vi "Process.vi"(8 "error in":errorcluster, 11 "Oxford1820 UI in":refnum<class "Instrument.Oxford1820 UI.lvclass">) -> (0 "error out":errorcluster, 3 "Oxford1820 UI out":refnum<class "Instrument.Oxford1820 UI.lvclass">)   [LabVIEW 2016, in "Instrument.Oxford1820 UI.lvclass"]
doc: "---------------------------------------------------------------\nJKI State Machine Objects™\nhttp://jki.net/state-machine-objects/\nCopyright (C) 2005-2015, JKI <info@jki.net>\nALL RIGHTS RESERVEDJKI State Machine Objects (SMO) 1.0.0.5\nJKI - JKI\nCopyright (c) 2016, JKI"
uses:
  Instrument.Oxford1820 UI.lvclass
  C:/Program Files (x86)/National Instruments/LabVIEW 2016/vi.lib/JKI/JKI SMO/SMO/SMO.lvclass
  C:/Program Files (x86)/National Instruments/LabVIEW 2016/user.lib/LevyLab/Levylab Instruments/SMOs/Instrument UI/Instrument UI.lvclass
  C:/Program Files (x86)/National Instruments/LabVIEW 2016/vi.lib/JKI/JKI SMO/SMO.UI/SMO.UI.lvclass
  <vilib>/JKI/JKI SMO/SMO/Typedefs/Parent Call--Enum.ctl
  Instrument.Oxford1820/Instrument.Oxford1820.lvclass
  C:/Program Files (x86)/National Instruments/LabVIEW 2016/user.lib/LevyLab/Levylab Instruments/SMOs/Instrument/Instrument.lvclass
  <userlib>/LevyLab/Levylab Instruments/SMOs/Instrument UI/Instrument UI.lvclass/Instrument UI.ctl
  Instrument.Oxford1820/Typedefs/getAll.ctl
  Instrument.Oxford1820/Typedefs/Fill Mode-Combo.ctl
  <instrlib>/Mercury iXX/Public/Libraries/Magnet/Controls/Switch Heater.ctl
  <userlib>/LevyLab/Levylab Instruments/SMOs/Instrument/Instrument.lvclass
  <userlib>/LevyLab/Levylab Instruments/SMOs/Instrument UI/Instrument UI.lvclass
  <vilib>/JKI/JKI SMO/SMO/SMO.lvclass
  <vilib>/JKI/JKI SMO/SMO.UI/SMO.UI.lvclass
  <instrlib>/Mercury iXX/Public/Libraries/Magnet.lvlib
panel:
  in  "Open Target":dbl=100.0 format="%.1f (%%)"
  out "System Time (HH:MM:SS)":dbl=165.3592643737793 format="%<%I:%M:%S %p>T"
  out "LPF on":dbl format="%<%H:%M:%S>t"
  out "PS Heat on (HH:MM:SS)":dbl format="%<%H:%M:%S>t"
  out "ETA":dbl=3660699600.0 format="%<%I:%M:%S %p %m/%d/%Y>T"
  out "version":string="v20/10/28"
  out "Waveform Chart 2":T1(graph)
  out "N2 LEVEL":dbl format="%.0f %"
  in  "Window Maximize":bool
  in  "Window Minimize":bool
  out "Magnet Status 3":string="Status: Clamped"
  in  "Remote Mode":bool
  out "Sentinel":bool=TRUE
  out "Voltage Meter":dbl(knob) caption="Voltage (V)" scale=-10.0..10.0
  out "Current Meter":dbl(knob) caption="Voltage (V)" scale=-180.0..180.0
  out "Magnet Field Meter":dbl(knob) caption="Voltage (V)" scale=-20.0..20.0
  in  "Hold":bool
  in  "To Set":bool
  in  "Export":bool
  out "PSU Field":dbl format="%#.5f T"
  in  "Target Field (T)":dbl caption="Field" format="%.2f"
  out "Target Field (T)":dbl caption="Field" format="%.2f T"
  in  "Target Rate (T/min)":dbl=0.1 caption="Rate" min=0.0 max=1.0 format="%.2f"
  out "Target Rate (T/min)":dbl caption="Rate" format="%.2f T/min"
  out "Field":dbl format="%.5f T"
  out "He LEVEL":dbl format="%.0f %"
  in  "PS Heat":bool
  in  "To Zero":bool
  in  "Clamp":bool
  out "N2 LVL":dbl format="%.1f (%%)"
  out "He LVL Chart":dbl(slide)=52.0833 scale=0.0..100.0
  out "N2 LVL Chart":dbl(slide)=61.3025 scale=0.0..100.0
  out "He LVL":dbl format="%.1f (%%)"
  in  "Fast/Slow Fill":bool
  in  "Open Needle Valve":bool
  in  "Close Needle Valve":bool
  in  "LPF Power":bool
  out "Needle Valve":dbl format="%.1f (%%)"
  out "Pressure":dbl format="%_5f mB"
  out "Magnet T":dbl format="%_2f K"
  out "Magnet R":dbl format="%_3f ohms"
  out "Voltage":dbl format="%.5f V"
  out "Current":dbl format="%.5f A"
  out "Magnet Status 2":string="Status: Clamped"
  in  "Power":bool
  # "Obsolete controls?"
  # "Actions"
  # "Targets"
  # "Status"
  # "Slow Rates\nCurrent Range (A)     Field Range (T)  Rate (T/min)\n0       -- 100        0    -- 11.5     0.91\n100     -- 150        11.5 -- 17.2     0.23\n150     -- 155.467    17.2 -- 18       0.11\n155.567 -- 172.471    18   -- 20       0.11\n\nFast Rates\nCurrent Range (A)     Field Range (T)  Rate (T/min)\n0       -- 155.467    0    -- 18       1.0\n155.567 -- 172.471    18   -- 20       0.25"
  # "IPS"
  # "PS Switch"
  # "Level"
  # "Level Graph"
  # "LPF"
  # "Helium"
  # "Nitrogen"
  # "^^^^"
  # "Needle Valve"
  # "Slow Rates\nCurrent Range (A)     Field Range (T)   Rate (T/min)\n0       -- 100        0    -- 11.5      0.91\n100     -- 150        11.5 -- 17.2      0.23\n150     -- 155.467    17.2 -- 18        0.11\n155.567 -- 172.471    18   -- 20        0.11\n\nFast Rates\nCurrent Range (A)     Field Range (T)   Rate (T/min)\n0       -- 155.467    0    -- 18        1.0\n155.567 -- 172.471    18   -- 20        0.25"
  # "SMO UI Template"
  # "For instructions on how to use the JKI State Machine Objects, examples and video tutorials, visit:\nhttp://jki.net/state-machine-objects/\n\nJKI State Machine Objects™\nhttp://jki.net/state-machine-objects/\nCopyright (C) 2005-2015, JKI <info@jki.net>\nALL RIGHTS RESERVED"
  # "Voltage (V)"
  # "Current (A)"
  # "Magnet (T)"
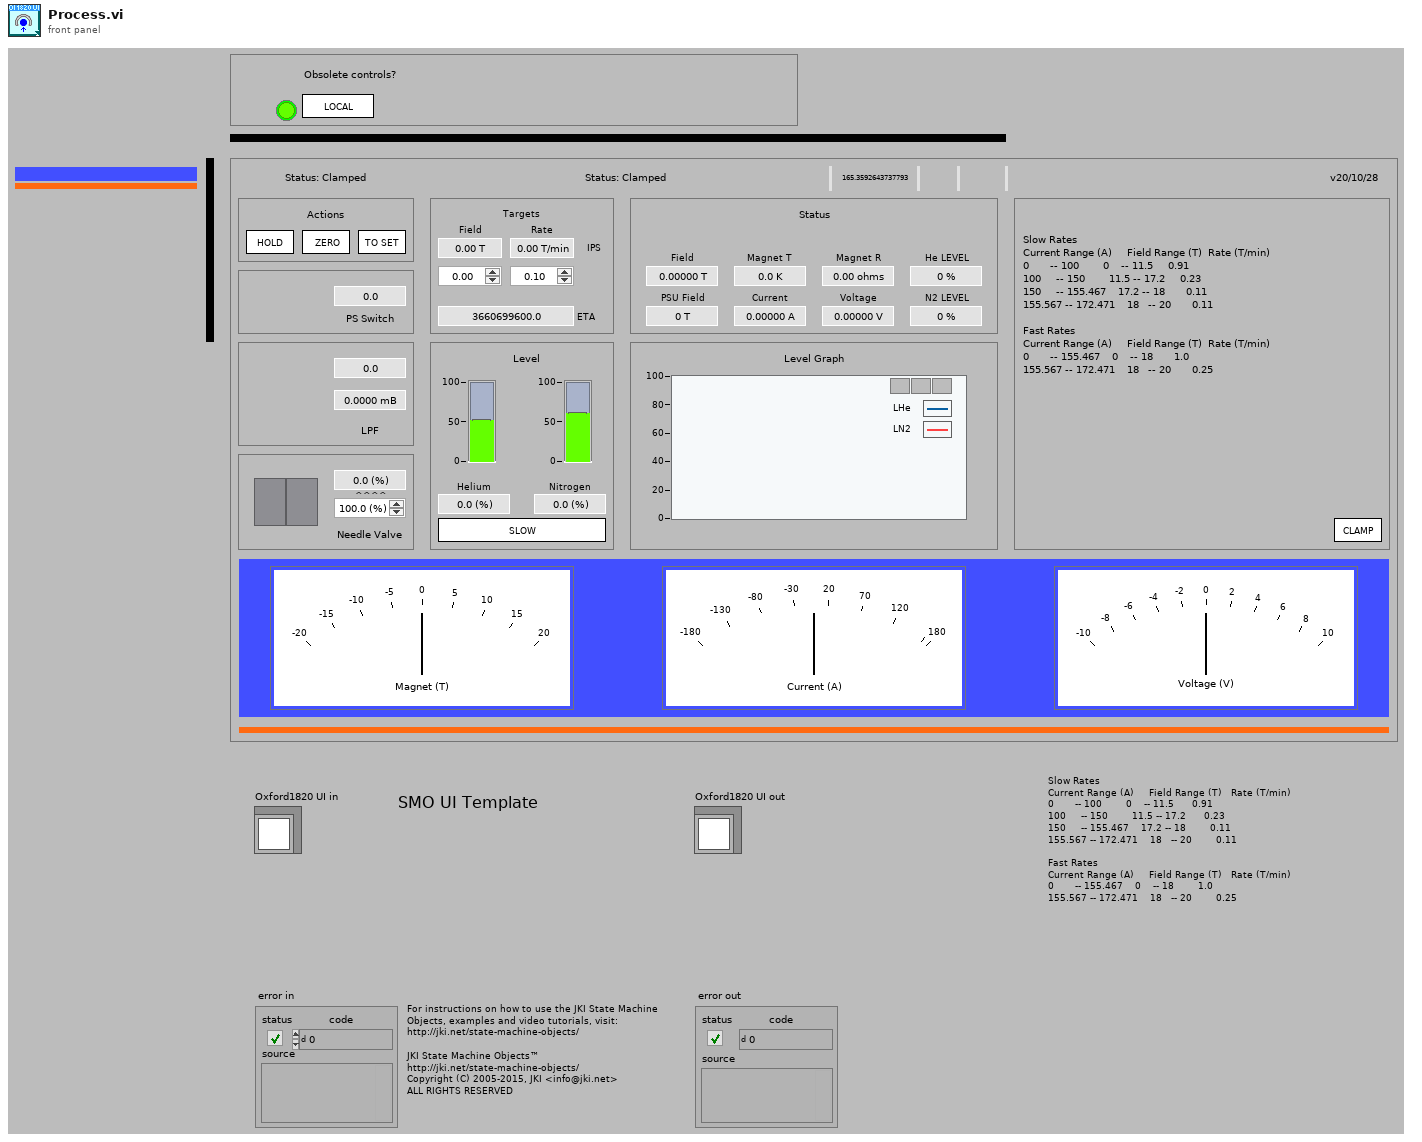
[diagram p1: front panel]
types:
  T1 = cluster{"1820_IPS_Level_He":dbl, "1820_IPS_Level_N2":dbl}
  T2 = typedef "SMO.lvclass/Parent Call--Enum.ctl" = enum16{"Allows parent to run", "Does not request parent to run"}
  T3 = enum32{"invalid app kind", "Development System", "Run Time System", "Student Edition", "Embedded LabVIEW", "Evaluation", "Custom"}
  T4 = typedef "Instrument.Oxford1820.lvclass/getAll.ctl" = cluster{"1820_IPS_Magnet_Field":dbl, "1820_IPS_PS_Field":dbl, "1820_IPS_Target_Field":dbl, "1820_IPS_Target_Field_Rate":dbl, "1820_IPS_Voltage":dbl, "1820_IPS_Current":dbl, "1820_IPS_Level_N2":dbl, "1820_IPS_Level_He":dbl, "1820_IPS_Magnet_Temperature":dbl, "1820_IPS_Magnet_Temperature_R":dbl, "1820_IPS_M1_Current":dbl, "1820_IPS_M1_Voltage":dbl, "1820_IPS_M2_Current":dbl, "1820_IPS_M2_Voltage":dbl, "1820_IPS_M3_Current":dbl, "1820_IPS_M3_Voltage":dbl, "1820_IPS_Status":string, "1820_IPS_Switch":string, "1820_ITC_Lambda_Temperature":dbl, "1820_ITC_Lambda_Temperature_R":dbl, "1820_ITC_Pressure":dbl, "1820_ITC_Needle_Valve":dbl}
  T5 = enum32{"Invalid", "Standard", "Closed", "Hidden", "Minimized", "Maximized"}
  T6 = typedef "Instrument.Oxford1820.lvclass/Fill Mode-Combo.ctl" = string
  T7 = typedef "Mercury iXX.lvlib/Magnet.lvlib/Switch Heater.ctl" = string
  T8 = typedef "RemoteControl.lvclass/Message--Cluster.ctl" = cluster{"Command":string, "Data":variant, "Message ID":i32}
  T9 = cluster{"Core":cluster{"Current VI Reference":refnum<vi>, "Close Panel on Exit?":bool, "error":errorcluster}, "Instrument UI out":refnum<class "Instrument.Oxford1820 UI.lvclass">, "Instrument":refnum<class "Instrument.Oxford1820.lvclass">, "getAll":variant, "Response":string, "config":variant, "switch time":timestamp, "LPF time":timestamp}
  T10 = cluster{"Current VI Reference":refnum<vi>, "Close Panel on Exit?":bool, "error":errorcluster}
  T11 = typedef "LVRectTypeDef.ctl" = cluster{"Left":i16, "Top":i16, "Right":i16, "Bottom":i16}
  T12 = typedef "SMO.lvclass/Protected Events.ctl" = cluster{"StopProcesses":refnum<user-event>, "AbortProcesses":refnum<user-event>, "Config Changed":refnum<user-event>, "Dependency":refnum<user-event>}
  T13 = typedef "Instrument.lvclass/PublicEvents--Cluster.ctl" = cluster{"MessageFromProcess":refnum<user-event>}
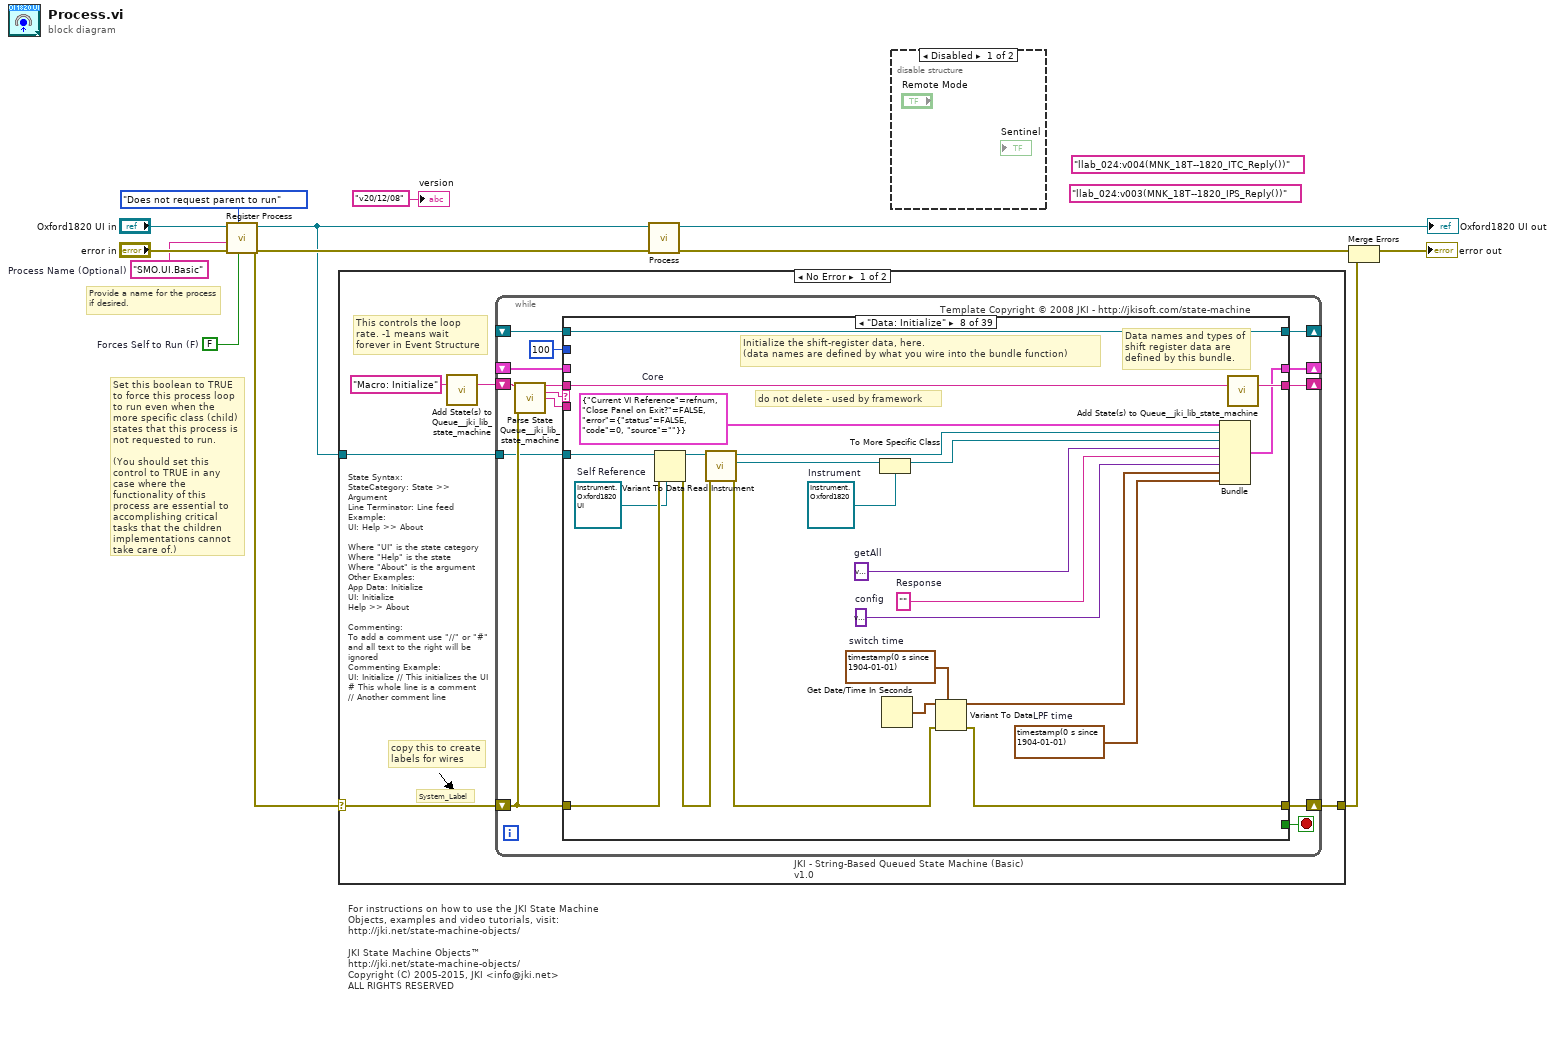
[diagram p0: block diagram]
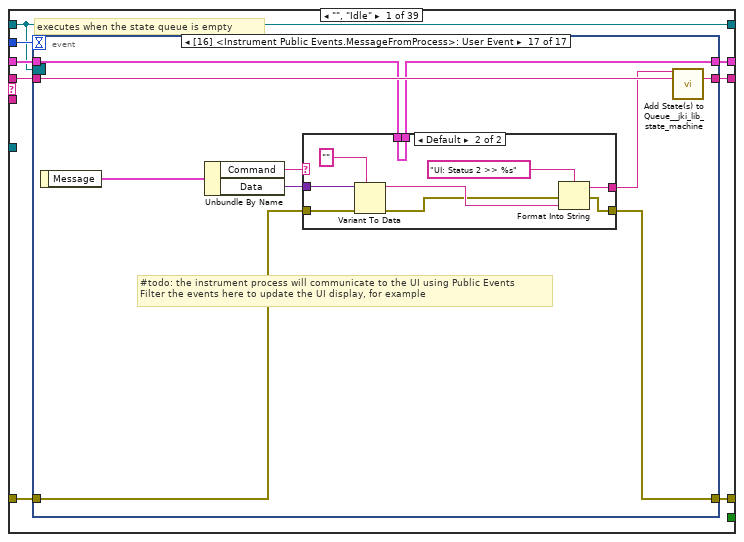
[diagram p3: hidden frame]
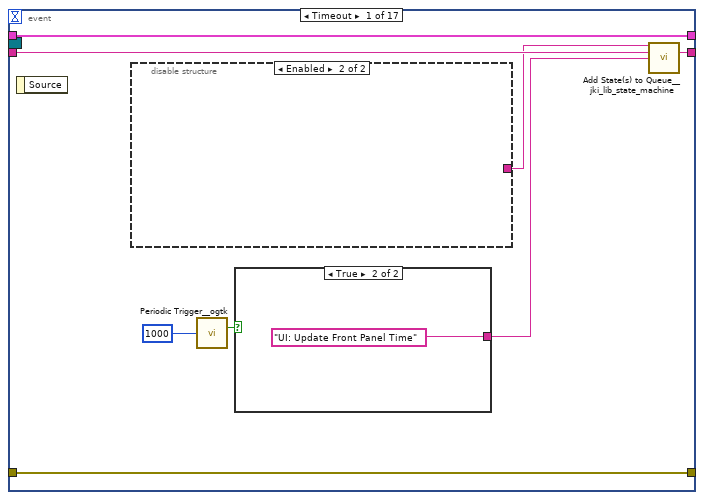
[diagram p4: hidden frame]
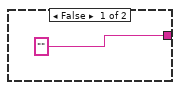
[diagram p5: hidden frame]
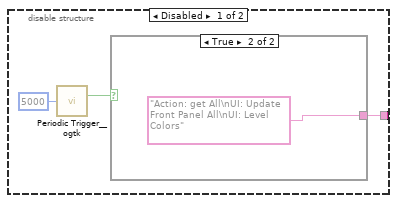
[diagram p6: hidden frame]
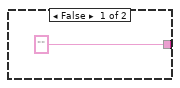
[diagram p7: hidden frame]
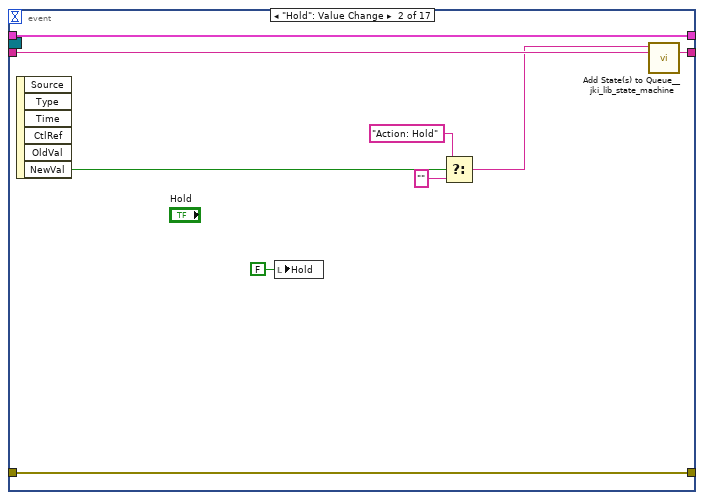
[diagram p8: hidden frame]
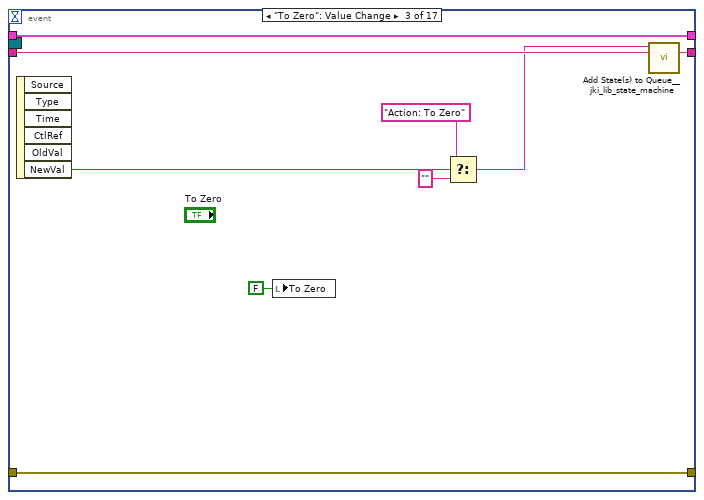
[diagram p9: hidden frame]
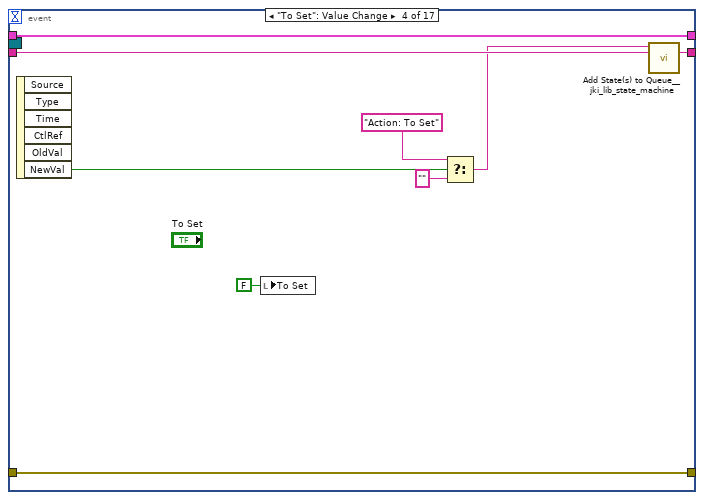
[diagram p10: hidden frame]
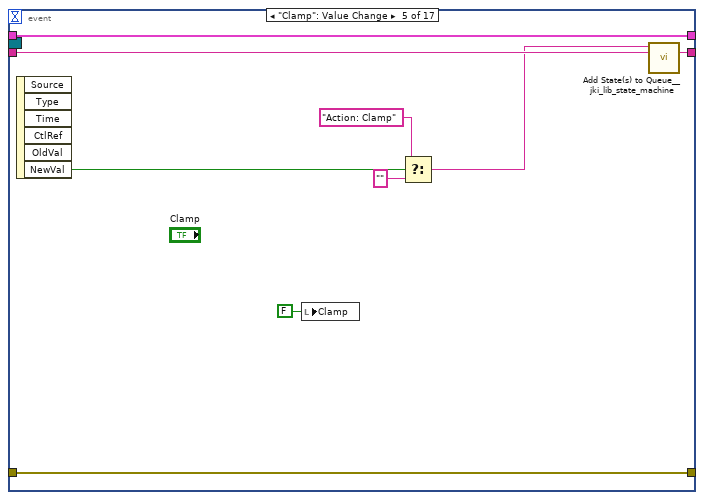
[diagram p11: hidden frame]
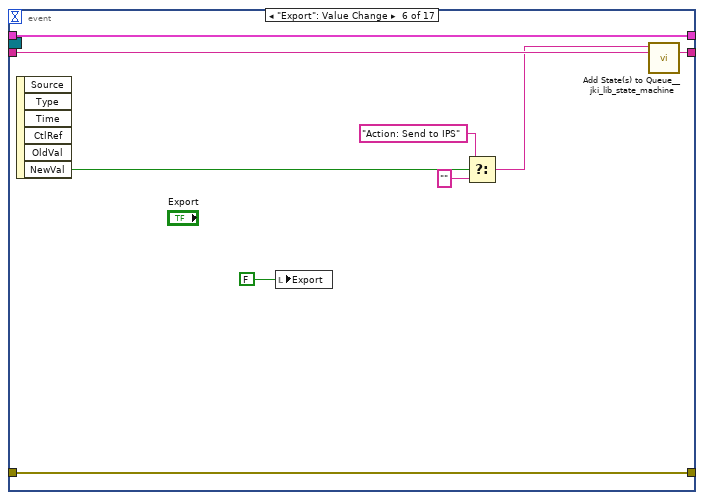
[diagram p12: hidden frame]
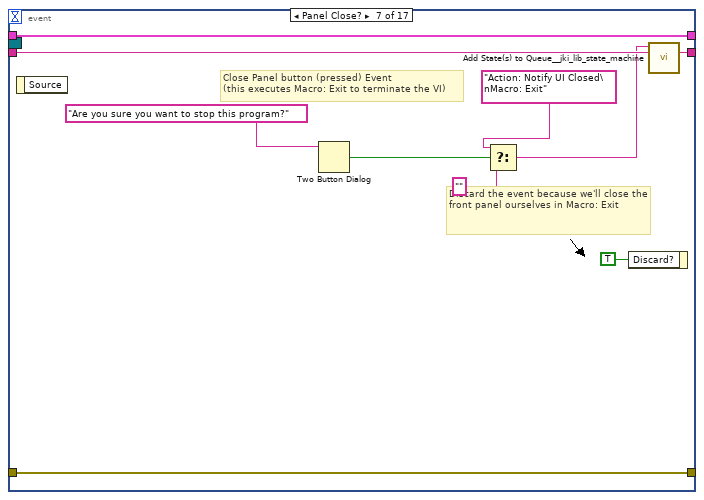
[diagram p13: hidden frame]
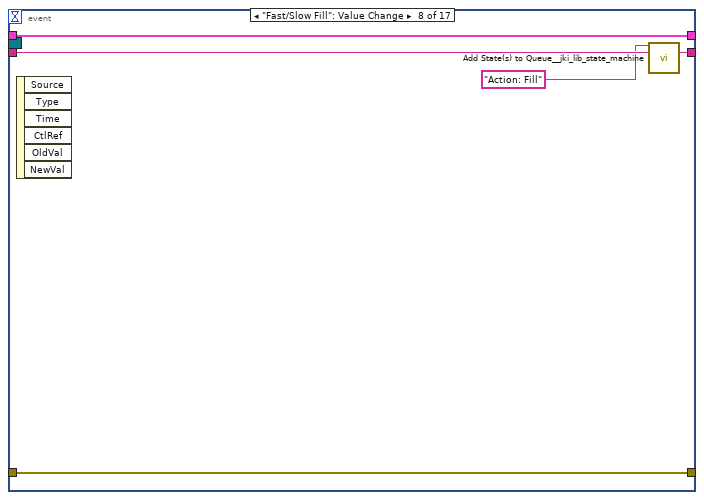
[diagram p14: hidden frame]
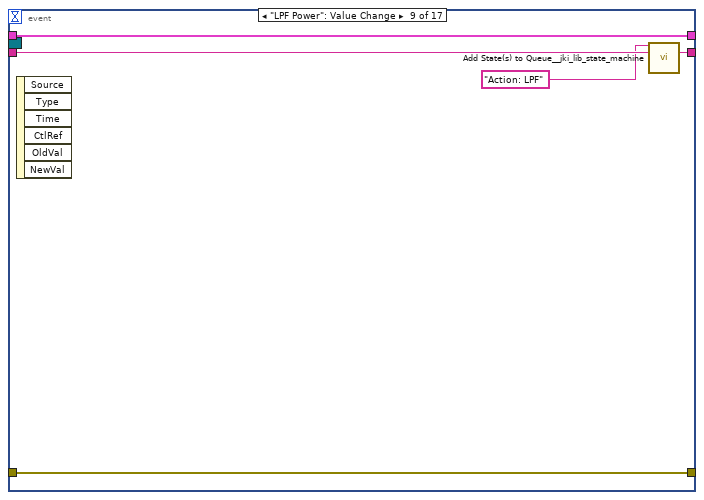
[diagram p15: hidden frame]
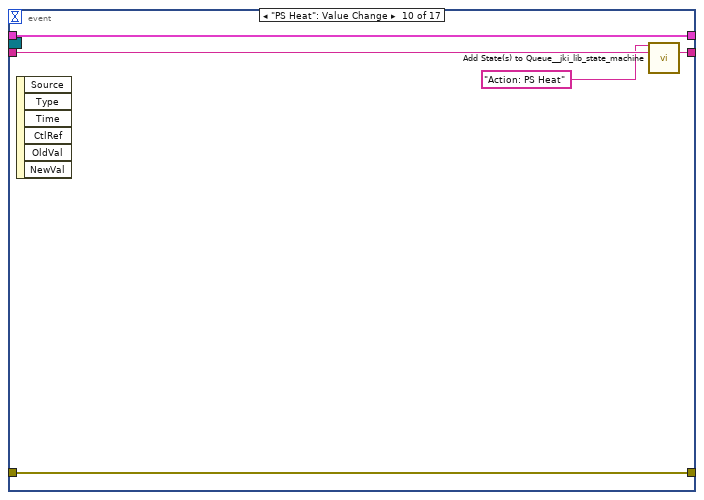
[diagram p16: hidden frame]
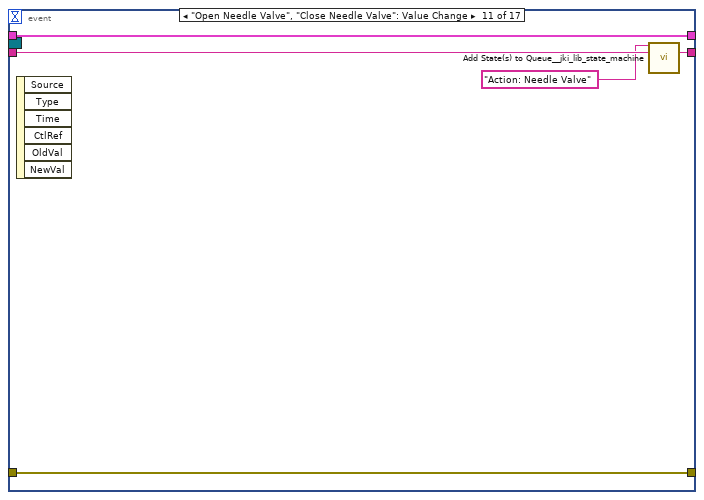
[diagram p17: hidden frame]
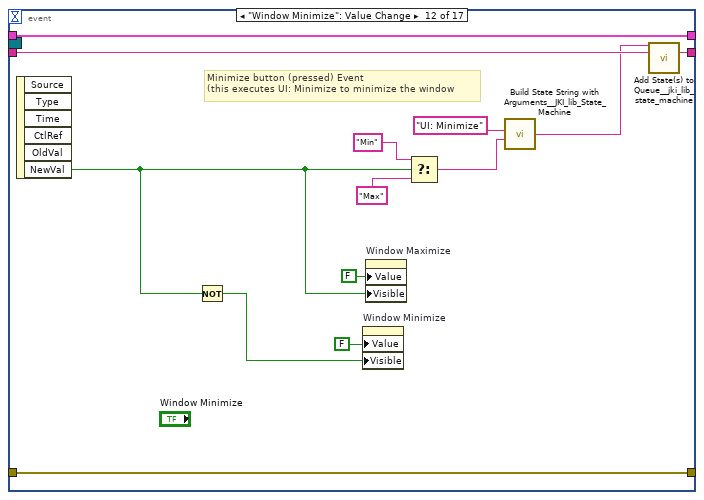
[diagram p18: hidden frame]
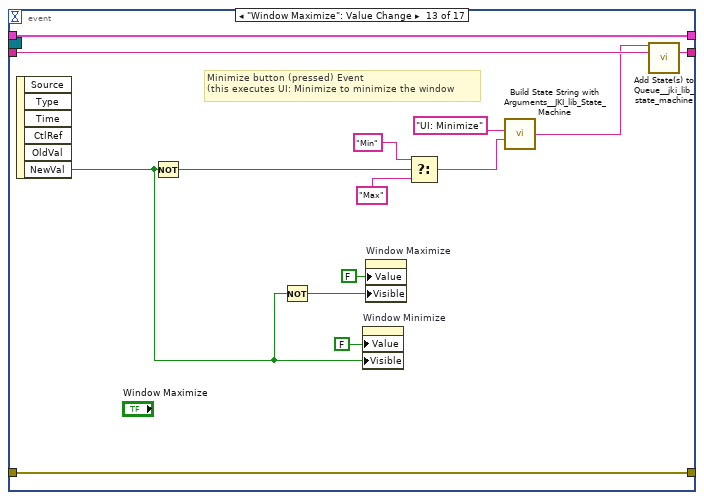
[diagram p19: hidden frame]
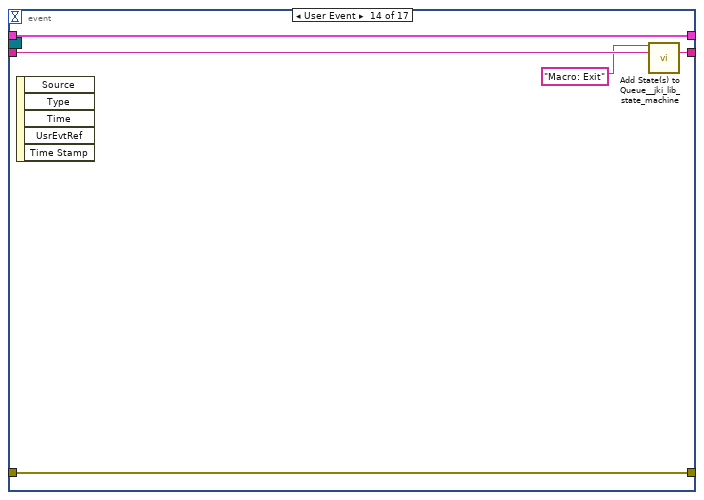
[diagram p20: hidden frame]
diagram:
  (unwired) "llab_024:v004(MNK_18T--1820_ITC_Reply())" ("variable")
  (unwired) "llab_024:v003(MNK_18T--1820_IPS_Reply())" ("variable")
  w3 = FALSE  # Forces Self to Run (F)
  w2 = "SMO.UI.Basic"  # Process Name (Optional)
  # "Provide a name for the process\nif desired."
  # "Set this boolean to TRUE to force this process loop to run even when the more specific class (child) states that this process is not requested to run.\n\n(You should set this control to TRUE in any case where the functionality of this process are essential to accomplishing critical tasks that the children implementations cannot take care of.)"
  # "For instructions on how to use the JKI State Machine Objects, examples and video tutorials, visit:\nhttp://jki.net/state-machine-objects/\n\nJKI State Machine Objects™\nhttp://jki.net/state-machine-objects/\nCopyright (C) 2005-2015, JKI <info@jki.net>\nALL RIGHTS RESERVED"
  n1 = call <vilib>:"Register Process.vi"("Forces Self to Run (F)"=w3, "Parent Call"=Parent_Call--Enum."Does not request parent to run", "error in (no error)"="error in", "Process Name (optional)"=w2, "SMO"="Oxford1820 UI in") -> ("error out"=w9:errorcluster, "SMO out"=w8:refnum<class "Instrument.Oxford1820 UI.lvclass">)  [unwired: 5 in]
  n2 = case shown="No Error" w9 {
    selector: w9 -> [w14 w628]
    tunnel: w8 -> [w15 _]
    tunnel: [w13 w628] -> w5
    frame No Error {
      # "State Syntax:\nStateCategory: State >> Argument\nLine Terminator: Line feed\nExample:\nUI: Help >> About\n\nWhere \"UI\" is the state category\nWhere \"Help\" is the state\nWhere \"About\" is the argument\nOther Examples:\nApp Data: Initialize\nUI: Initialize\nHelp >> About\n\nCommenting:\nTo add a comment use \"//\" or \"#\" and all text to the right will be ignored\nCommenting Example:\nUI: Initialize // This initializes the UI\n# This whole line is a comment\n// Another comment line"
      # "copy this to create labels for wires"
      # "This controls the loop rate. -1 means wait forever in Event Structure"
      # "System_Label"
      n3 = call <vilib>:"Add State(s) to Queue__jki_lib_state_machine.vi"("State(s) in (\"\")"="Macro: Initialize") -> ("States Out"=w17:string)  [unwired: 14 in]
      n4 = while "JKI - String-Based Queued State Machine (Basic) v1.0" {
        shift-right: [w24] -> _
        shift-left: _ -> [w23]
        shift-right: [w27] -> w13
        shift-left: w14 -> [w21]
        shift-right: [w26] -> _
        shift-left: w17 -> [w28]
        tunnel: w15 -> [w20]
        shift-right: [w19] -> _
        shift-left: _ -> [w18]
        stop <- w25 stop-if-true
        # "Template Copyright © 2008 JKI - http://jkisoft.com/state-machine"
        n5 = call <vilib>:"Parse State Queue__jki_lib_state_machine.vi"("State Queue"=w28, "Error In (no error)"=w21) -> ("Remaining States"=w30:string, "Current State"=w31:string, "Arguments"=w29:string)  [unwired: 11 in]
        n6 = case shown="\"Data: Initialize\"" w31 {
          selector: w31 -> [_ _ w206 _ _ _ _ _ _ _ _ _ _ _ _ _ _ _ _ _ _ _ _ _ _ _ _ _ _ _ _ _ _ _ _ _ _ _ _]
          tunnel: w30 -> [w39 w204 w210 w229 w243 w249 w254 w277 w284 w289 w300 w326 w344 w350 w357 w364 w380 w414 w440 w449 w463 w468 w479 w486 w491 w505 w511 w518 w525 w535 w542 w549 w556 w563 w574 w587 w600 w618 w627]
          tunnel: w29 -> [_ _ _ _ _ _ _ _ _ _ _ _ _ w345 _ w358 w374 w415 _ _ _ _ _ _ _ _ _ _ _ _ _ _ _ _ _ _ _ _ _]
          tunnel: w23 -> [w37 w201 w208 w220 w231 w245 w251 _ w279 w286 w298 w323 w340 w347 w354 w362 w376 w413 w437 w445 w454 w465 w476 w481 w488 w503 w509 w514 w521 w526 w539 w546 w553 w557 w571 w577 w597 w609 w624]
          tunnel: [w36 w202 w212 w226 w236 w244 w252 w265 w280 w287 w295 w321 w342 w348 w355 w359 w377 w408 w438 w447 w461 w466 w470 w482 w489 w499 w506 w515 w519 w529 w536 w543 w550 w558 w568 w582 w588 w614 w621] -> w27
          tunnel: w21 -> [w35 w202 w211 w226 w232 _ w252 w274 w281 w287 w296 w322 w342 w348 w355 w360 w378 w409 w438 w447 w461 w466 w471 w483 w489 w494 w507 w515 w520 w530 w537 w544 w551 w559 w569 w583 w595 w615 w622]
          tunnel: [w38 w203 w209 w228 w242 w248 w253 w276 w283 w288 w299 w325 w343 w349 w356 w363 w379 w419 w439 w448 w462 w467 w478 w485 w490 w504 w510 w517 w524 w534 w541 w548 w555 w562 w573 w586 w599 w617 w626] -> w26
          tunnel: [_ _ _ _ _ TRUE _ _ _ _ _ _ _ _ _ _ _ _ _ _ _ _ _ _ _ _ _ _ _ _ _ _ _ _ _ _ _ _ _] -> w25
          tunnel: [w34 w201 w208 w227 w234 w245 w251 w275 w279 w286 w298 w323 w340 w347 w354 w362 w376 w413 w437 w445 w454 w465 w476 w481 w488 w503 w509 w513 w521 w532 w539 w546 w553 w557 w571 w576 w597 w607 w624] -> w24
          tunnel: 100 ("Timeout") -> [w33 _ _ _ _ _ _ _ _ _ _ _ _ _ _ _ _ _ _ _ _ _ _ _ _ _ _ _ _ _ _ _ _ _ _ _ _ _ _]
          tunnel: w20 -> [_ _ _ _ _ _ _ w262 _ _ _ _ _ _ _ _ _ _ _ _ _ _ _ _ _ _ _ _ _ _ _ _ _ _ _ _ _ _ _]
          tunnel: [w32 w200 w205 w217 w241 w246 w250 w272 w278 w285 w297 w324 w341 w346 w353 w361 w373 w418 w436 w446 w455 w464 w477 w484 w487 w502 w508 w516 w523 w533 w540 w547 w554 w561 w572 w585 w598 w616 w625] -> w19
          tunnel: w18 -> [w32 w200 w205 w217 w241 w246 w250 w272 w278 w285 w297 w324 w341 w346 w353 w361 w373 w418 w436 w446 w455 w464 w477 w484 w487 _ w508 w516 w523 w533 w540 w547 w554 w561 w572 w585 w598 w616 w625]
          frame "", "Idle" {
            # "executes when the state queue is empty"
            n7 = event shown="[16] <Instrument Public Events.MessageFromProcess>: User Event" {
              selector: w32 -> [_ _ _ _ _ _ _ _ _ _ _ _ _ _ _ _ _]
              dyn-events: _ -> [_ _ _ _ _ _ _ _ _ _ _ _ _ _ _ _ _]
              timeout: w33 -> [_ _ _ _ _ _ _ _ _ _ _ _ _ _ _ _ _]
              tunnel: w39 -> [w47 w63 w72 w81 w90 w99 w109 w114 w119 w124 w129 w142 w156 w161 w166 w175 w185]
              tunnel: [w46 w62 w71 w80 w89 w98 w108 w113 w118 w123 w128 w141 w155 w160 w165 w174 w184] -> w38
              tunnel: w37 -> [w43 w60 w69 w78 w87 w96 w106 w112 w117 w122 w127 w140 w154 w158 w163 w172 w183]
              tunnel: [w45 w61 w70 w79 w88 w97 w105 w111 w116 w121 w126 w139 w153 w159 w164 w173 w176] -> w36
              tunnel: w35 -> [w45 w61 w70 w79 w88 w97 w105 w111 w116 w121 w126 w139 w153 w159 w164 w173 w177]
              tunnel: [w43 w60 w69 w78 w87 w96 w106 w112 w117 w122 w127 w140 w154 w158 w163 w172 w182] -> w34
              event Timeout {
                n8 = event-data() -> ()  [unwired: 1 in, 1 out]
                n9 = disable-structure shown="Enabled" {
                  disable-tunnel: [w50 _] -> w44
                  frame Disabled {
                    n10 = call <userlib>:"Periodic Trigger__ogtk.vi"("time (ms)"=u32 5000 ("update time (ms)")) -> ("Triggered"=w52:bool)  [unwired: 12 in, 2 out]
                    n11 = case shown="True" w52 {
                      tunnel: ["" "Action: get All\nUI: Update Front Panel All\nUI: Level Colors"] -> w50
                      frame False {
                      }
                      frame True {
                      }
                    }
                  }
                  frame Enabled {
                  }
                }
                n12 = call <userlib>:"Periodic Trigger__ogtk.vi"("time (ms)"=u32 1000 ("update time (ms)")) -> ("Triggered"=w41:bool)  [unwired: 12 in, 2 out]
                n13 = case shown="True" w41 {
                  tunnel: ["" "UI: Update Front Panel Time"] -> w40
                  frame False {
                  }
                  frame True {
                  }
                }
                n14 = call <vilib>:"Add State(s) to Queue__jki_lib_state_machine.vi"("State(s) in Front (\"\")"=w44, "State(s) in (\"\")"=w47, "State(s) at Back (\"\")"=w40) -> ("States Out"=w46:string)  [unwired: 12 in]
              }
              event "Hold": Value Change {
                n15 = event-data() -> ("NewVal"=w59:bool)  [unwired: 1 in, 5 out]
                n16 = local write "Hold"(FALSE ("Hold")) -> ()
                n17 = Select(t="Action: Hold" ("State(s) in Front (\"\")"), s=w59, f="") -> (s? t:f=w56:string)
                n18 = call <vilib>:"Add State(s) to Queue__jki_lib_state_machine.vi"("State(s) in Front (\"\")"=w56, "State(s) in (\"\")"=w63) -> ("States Out"=w62:string)  [unwired: 13 in]
              }
              event "To Zero": Value Change {
                n19 = event-data() -> ("NewVal"=w67:bool)  [unwired: 1 in, 5 out]
                n20 = local write "To Zero"(FALSE ("To Zero")) -> ()
                n21 = Select(t="Action: To Zero" ("State(s) in Front (\"\")"), s=w67, f="") -> (s? t:f=w65:string)
                n22 = call <vilib>:"Add State(s) to Queue__jki_lib_state_machine.vi"("State(s) in Front (\"\")"=w65, "State(s) in (\"\")"=w72) -> ("States Out"=w71:string)  [unwired: 13 in]
              }
              event "To Set": Value Change {
                n23 = event-data() -> ("NewVal"=w76:bool)  [unwired: 1 in, 5 out]
                n24 = local write "To Set"(FALSE ("To Set")) -> ()
                n25 = Select(t="Action: To Set" ("State(s) in Front (\"\")"), s=w76, f="") -> (s? t:f=w74:string)
                n26 = call <vilib>:"Add State(s) to Queue__jki_lib_state_machine.vi"("State(s) in Front (\"\")"=w74, "State(s) in (\"\")"=w81) -> ("States Out"=w80:string)  [unwired: 13 in]
              }
              event "Clamp": Value Change {
                n27 = event-data() -> ("NewVal"=w85:bool)  [unwired: 1 in, 5 out]
                n28 = local write "Clamp"(FALSE ("Clamp")) -> ()
                n29 = Select(t="Action: Clamp" ("State(s) in Front (\"\")"), s=w85, f="") -> (s? t:f=w83:string)
                n30 = call <vilib>:"Add State(s) to Queue__jki_lib_state_machine.vi"("State(s) in Front (\"\")"=w83, "State(s) in (\"\")"=w90) -> ("States Out"=w89:string)  [unwired: 13 in]
              }
              event "Export": Value Change {
                n31 = event-data() -> ("NewVal"=w95:bool)  [unwired: 1 in, 5 out]
                n32 = local write "Export"(FALSE ("Send to IPS")) -> ()
                n33 = Select(t="Action: Send to IPS" ("State(s) in Front (\"\")"), s=w95, f="") -> (s? t:f=w92:string)
                n34 = call <vilib>:"Add State(s) to Queue__jki_lib_state_machine.vi"("State(s) in Front (\"\")"=w92, "State(s) in (\"\")"=w99) -> ("States Out"=w98:string)  [unwired: 13 in]
              }
              event Panel Close? {
                # "Discard the event because we'll close the front panel ourselves in Macro: Exit"
                # "Close Panel button (pressed) Event\n(this executes Macro: Exit to terminate the VI)"
                n35 = event-data() -> ()  [unwired: 1 in, 1 out]
                n36 = Two Button Dialog(message="Are you sure you want to stop this program?") -> (T button?=w104:bool)  [unwired: 2 in]
                n37 = Select(t="Action: Notify UI Closed\nMacro: Exit", s=w104, f="") -> (s? t:f=w100:string)
                n38 = event-data("Discard?"=TRUE) -> ()  [unwired: 1 in, 1 out]
                n39 = call <vilib>:"Add State(s) to Queue__jki_lib_state_machine.vi"("State(s) in Front (\"\")"=w100, "State(s) in (\"\")"=w109) -> ("States Out"=w108:string)  [unwired: 13 in]
              }
              event "Fast/Slow Fill": Value Change {
                n40 = event-data() -> ()  [unwired: 1 in, 6 out]
                n41 = call <vilib>:"Add State(s) to Queue__jki_lib_state_machine.vi"("State(s) in Front (\"\")"="Action: Fill", "State(s) in (\"\")"=w114) -> ("States Out"=w113:string)  [unwired: 13 in]
              }
              event "LPF Power": Value Change {
                n42 = event-data() -> ()  [unwired: 1 in, 6 out]
                n43 = call <vilib>:"Add State(s) to Queue__jki_lib_state_machine.vi"("State(s) in Front (\"\")"="Action: LPF", "State(s) in (\"\")"=w119) -> ("States Out"=w118:string)  [unwired: 13 in]
              }
              event "PS Heat": Value Change {
                n44 = event-data() -> ()  [unwired: 1 in, 6 out]
                n45 = call <vilib>:"Add State(s) to Queue__jki_lib_state_machine.vi"("State(s) in Front (\"\")"="Action: PS Heat", "State(s) in (\"\")"=w124) -> ("States Out"=w123:string)  [unwired: 13 in]
              }
              event "Open Needle Valve", "Close Needle Valve": Value Change {
                n46 = event-data() -> ()  [unwired: 1 in, 6 out]
                n47 = call <vilib>:"Add State(s) to Queue__jki_lib_state_machine.vi"("State(s) in Front (\"\")"="Action: Needle Valve", "State(s) in (\"\")"=w129) -> ("States Out"=w128:string)  [unwired: 13 in]
              }
              event "Window Minimize": Value Change {
                # "Minimize button (pressed) Event\n(this executes UI: Minimize to minimize the window"
                n48 = event-data() -> ("NewVal"=w130:bool)  [unwired: 1 in, 5 out]
                n49 = Not(x=w130) -> (.not. x?=w131:bool)
                n50 = property on="Window Minimize" class="Bool (strict)"("Value"=FALSE ("Window Maximize"), "Visible"=w131) -> ()  [unwired: 2 in, 2 out]
                n51 = property on="Window Maximize" class="Bool (strict)"("Value"=FALSE ("Window Maximize"), "Visible"=w130) -> ()  [unwired: 2 in, 2 out]
                n52 = Select(t="Min" ("Arguments (\"\")"), s=w130, f="Max" ("Arguments (\"\")")) -> (s? t:f=w135:string)
                n53 = call <vilib>:"Build State String with Arguments__JKI_lib_State_Machine.vi"("Arguments (\"\")"=w135, "State"="UI: Minimize") -> ("State with Arguments"=w134:string)  [unwired: 4 in]
                n54 = call <vilib>:"Add State(s) to Queue__jki_lib_state_machine.vi"("State(s) in Front (\"\")"=w134, "State(s) in (\"\")"=w142) -> ("States Out"=w141:string)  [unwired: 13 in]
              }
              event "Window Maximize": Value Change {
                # "Minimize button (pressed) Event\n(this executes UI: Minimize to minimize the window"
                n55 = event-data() -> ("NewVal"=w144:bool)  [unwired: 1 in, 5 out]
                n56 = Not(x=w144) -> (.not. x?=w145:bool)
                n57 = Not(x=w144) -> (.not. x?=w143:bool)
                n58 = property on="Window Minimize" class="Bool (strict)"("Value"=FALSE ("Window Maximize"), "Visible"=w144) -> ()  [unwired: 2 in, 2 out]
                n59 = property on="Window Maximize" class="Bool (strict)"("Value"=FALSE ("Window Maximize"), "Visible"=w143) -> ()  [unwired: 2 in, 2 out]
                n60 = Select(t="Min" ("Arguments (\"\")"), s=w145, f="Max" ("Arguments (\"\")")) -> (s? t:f=w149:string)
                n61 = call <vilib>:"Build State String with Arguments__JKI_lib_State_Machine.vi"("Arguments (\"\")"=w149, "State"="UI: Minimize") -> ("State with Arguments"=w148:string)  [unwired: 4 in]
                n62 = call <vilib>:"Add State(s) to Queue__jki_lib_state_machine.vi"("State(s) in Front (\"\")"=w148, "State(s) in (\"\")"=w156) -> ("States Out"=w155:string)  [unwired: 13 in]
              }
              event User Event {
                n63 = event-data() -> ()  [unwired: 1 in, 5 out]
                n64 = call <vilib>:"Add State(s) to Queue__jki_lib_state_machine.vi"("State(s) in Front (\"\")"="Macro: Exit", "State(s) in (\"\")"=w161) -> ("States Out"=w160:string)  [unwired: 13 in]
              }
              event User Event {
                # "On Abort, no nice macro exit, but exit right away"
                n65 = event-data() -> ()  [unwired: 1 in, 5 out]
                n66 = call <vilib>:"Add State(s) to Queue__jki_lib_state_machine.vi"("State(s) in Front (\"\")"="Exit", "State(s) in (\"\")"=w166) -> ("States Out"=w165:string)  [unwired: 13 in]
              }
              event "Power": Value Change {
                # "if user pushes stop button, give them a window to make sure they\nmeant to stop this program"
                n67 = event-data() -> ()  [unwired: 1 in, 6 out]
                n68 = Two Button Dialog(message="Are you sure you want to stop this program?") -> (T button?=w171:bool)  [unwired: 2 in]
                n69 = Select(t="Macro: Exit", s=w171, f="") -> (s? t:f=w167:string)
                n70 = call <vilib>:"Add State(s) to Queue__jki_lib_state_machine.vi"("State(s) in Front (\"\")"=w167, "State(s) in (\"\")"=w175) -> ("States Out"=w174:string)  [unwired: 13 in]
              }
              event User Event {
                # "#todo: the instrument process will communicate to the UI using Public Events\nFilter the events here to update the UI display, for example"
                n71 = event-data() -> ("Message"=w178:T8)  [unwired: 1 in]
                n72 = Unbundle By Name(w178) -> ("Command"=w180:string, "Data"=w181:variant)
                n73 = case shown="Default" w180 {
                  tunnel: w181 -> [w190 w198]
                  tunnel: w183 -> [w189 w199]
                  tunnel: [w188 w199] -> w182
                  tunnel: ["UI: Update Front Panel All" w195] -> w179
                  tunnel: w177 -> [w186 w192]
                  tunnel: [w186 w191] -> w176
                  frame "getAll" {
                    n74 = Bundle By Name(cluster=w189, "getAll"=w190) -> (w188:T9)
                  }
                  frame Default {
                    n75 = Variant To Data(error in=w192, type="", Variant=w198) -> (data=w194:string, error out=w193:errorcluster)
                    n76 = Format Into String(format string="UI: Status 2 >> %s", error in=w193, w194) -> (resulting string=w195:string, error out=w191:errorcluster)  [unwired: 1 in]
                  }
                }
                n77 = call <vilib>:"Add State(s) to Queue__jki_lib_state_machine.vi"("State(s) in Front (\"\")"=w179, "State(s) in (\"\")"=w185) -> ("States Out"=w184:string)  [unwired: 13 in]
              }
            }
          }
          frame "---------- Core ----------" {
            # "Do not put any code in this frame.\n(it is a separator no-op)"
            n78 = call <vilib>:"Add State(s) to Queue__jki_lib_state_machine.vi"("State(s) in (\"\")"=w204) -> ("States Out"=w203:string)  [unwired: 14 in]
          }
          frame Default {
            w215 = 42 items=["No error", "Argument error", "Memory is full", "Out of zone", "End of file", "File already open", "Generic file I/O error", "File not found", "File permission error", "Disk is full", "Duplicate path", "Too many files open", "System feature not enabled", "Resource file not found", "Cannot add resource", "Resource not found", "Image not found", "Image memory error", "Pen does not exist", "Config type invalid", "Config token not found", "Config parse error", "Config memory error", "Bad external code format", "Bad external code offset", "External code not present", "Null window", "Destroy window error", "Null menu", "Print aborted", "Bad print record", "Print driver error", "Windows error during printing", "Memory error during printing", "Print dialog error", "Generic print error", "Invalid device refnum", "Device not found", "Device parameter error", "Device unit error", "Cannot open device", "Device call aborted", "Generic error", "Cancelled by user", "Object ID too low", "Object ID too high", "Object not in heap", "Unknown heap", "Unknown object (invalid DefProc)", "Unknown object (DefProc not in table)", "Message out of range", "Invalid (null) method", "Unknown message", "Manager call not supported", "Bad address", "Network operation in progress", "Network operation timed out", "Connection is busy", "Network attribute not supported", "Network error", "Address in use", "System out of memory", "Connection aborted", "Connection refused", "Not connected", "Already connected", "Connection closed", "Initialization error (interapplication manager)", "Bad occurrence", "Wait on unbound occurrence handler", "Occurrence queue overflow", "Datalog type conflict", "Unused", "Unrecognized type (interapplication manager)", "Memory corrupt", "Failed to make temporary DLL", "Old CIN version", "Drag socket not found", "Failed to load drop-object", "Failed to register OLE object", "Failed to release OLE object", "Format specifier type mismatch", "Unknown format specifier", "Too few format specifiers", "Too many format specifiers", "Scan failed", "Newer CIN version", "Error converting to variant", "Runtime menu error", "Password tampered", "Variant attribute not found", "Incompatible variant data type", "Event data is not available", "Event Store is not present", "Occurrence is not found", "Event Queue is not created", "Event info is not available", "Refnum passed is NULL", "Error retrieving Class GUID", "Error retrieving CoClass GUID", "Error retrieving TypeLib GUID.", "Bad built application magic bytes.", "Specific driver is different from the specific driver associated with the Logical Name.", "There is no session opened to the class driver.", "Max Error", "MAX - Error with config objects", "MAX - Error loading configuration", "MAX - Group not supported"]
            # "Current State"
            # "Do not delete, rename, or modify this frame.\n(this is used to capture unhandled states and typos)"
            # "Handle mistyped state name (developer tool)"
            n79 = Format Into String(format string="Software Exception: Unhandled State \"%s\"." ("message"), error in=w211, w206) -> (resulting string=w214:string, error out=w213:errorcluster)  [unwired: 1 in]
            n80 = call <vilib>:"Error Cluster From Error Code.vi"("show call chain? (False)"=TRUE, "error in (no error)"=w213, "error message (\"\")"=w214, "error code (0)"=w215) -> ("error out"=w212:errorcluster)  [unwired: 5 in]
            n81 = call <vilib>:"Add State(s) to Queue__jki_lib_state_machine.vi"("State(s) in (\"\")"=w210) -> ("States Out"=w209:string)  [unwired: 14 in]
          }
          frame "Initialize Core Data" {
            # "Do not delete, rename, or modify this frame.\n(this is used to determine panel behavior on exit)"
            # "originally closed?"
            # "exe?"
            # "If panel starts closed or is an EXE, then close it when we exit"
            n82 = property class="VI"() -> ("Front Panel.Open"=w225:bool)  [unwired: 2 in, 2 out]
            n83 = property class="App"() -> ("App.Kind"=w224:T3)  [unwired: 2 in, 2 out]
            n84 = control-ref of="Current VI Reference"() -> (w218:refnum<vi>)
            n85 = Not(x=w225) -> (.not. x?=w222:bool)
            n86 = Equal?(x=w224, y=T3."Run Time System" ("Application:Kind")) -> (x = y?=w221:bool)
            n87 = Or(x=w222, y=w221) -> (x .or. y?=w219:bool)
            n88 = Bundle By Name(cluster=w220, "Core.Current VI Reference"=w218, "Core.Close Panel on Exit?"=w219) -> (w227:T9)
            n89 = call <vilib>:"Add State(s) to Queue__jki_lib_state_machine.vi"("State(s) in (\"\")"=w229) -> ("States Out"=w228:string)  [unwired: 14 in]
          }
          frame "Error Handler" {
            w236 = errorcluster {"status"=FALSE, "code"=0, "source"=""}  # No error
            # "Overwrite this method to handle errors and pass to parent if not handled. Parent will fire a public event if the error is not handled up the chain of classes."
            # "Handle any errors here.\nYou can also output any states to clean-up after errors occur"
            n90 = Unbundle By Name(w231) -> ("Instrument UI out"=w240:refnum<class "Instrument.Oxford1820 UI.lvclass">)
            n91 = call-dynamic "Handle Error.vi"("Stop on Unhandled Error (T)"=FALSE, "error in"=w232, "Instrument.Oxford1820 UI"=w240) -> ("handling error"=w230:errorcluster, "Unhandled error"=w235:errorcluster)  [unwired: 6 in, 1 out]
            n92 = Bundle By Name(cluster=w231, "Core.error"=w235) -> (w234:T9)
            n93 = Select(t="Exit", s=w230, f="") -> (s? t:f=w237:string)
            n94 = call <vilib>:"Add State(s) to Queue__jki_lib_state_machine.vi"("State(s) in Front (\"\")"=w237, "State(s) in (\"\")"=w243) -> ("States Out"=w242:string)  [unwired: 13 in]
          }
          frame "Exit" {
            # "Do not put any code in this frame.\n(No errors that occur here will be handled.)"
            n95 = Unbundle By Name(w245) -> ("Core.error"=w244:errorcluster)
            n96 = call <vilib>:"Add State(s) to Queue__jki_lib_state_machine.vi"("State(s) in (\"\")"=w249) -> ("States Out"=w248:string)  [unwired: 14 in]
          }
          frame "---------- Data ----------" {
            # "Do not put any code in this frame.\n(It is a separator no-op. You can make a copy of this frame to create a new Data frame)"
            n97 = call <vilib>:"Add State(s) to Queue__jki_lib_state_machine.vi"("State(s) in (\"\")"=w254) -> ("States Out"=w253:string)  [unwired: 14 in]
          }
          frame "Data: Initialize" {
            w255 = refnum<class "Instrument.Oxford1820.lvclass"> refnum  # Instrument
            w263 = timestamp(0 s since 1904-01-01)  # LPF time
            w267 = timestamp(0 s since 1904-01-01)  # switch time
            w268 = variant  # config
            w269 = ""  # Response
            w270 = variant  # getAll
            w271 = T10 {"Current VI Reference"=refnum, "Close Panel on Exit?"=FALSE, "error"={"status"=FALSE, "code"=0, "source"=""}}  # Core
            w273 = refnum<class "Instrument.Oxford1820 UI.lvclass"> refnum  # Self Reference
            # "do not delete - used by framework"
            # "Data names and types of shift register data are defined by this bundle."
            # "Initialize the shift-register data, here.\n(data names are defined by what you wire into the bundle function)"
            n98 = Variant To Data(error in=w274, type=w273, Variant=w262) -> (data=w261:refnum<class "Instrument.Oxford1820 UI.lvclass">, error out=w260:errorcluster)
            n99 = call <userlib>:"Read Instrument.vi"("error in (no error)"=w260, "Instrument UI in"=w261) -> ("error out"=w259:errorcluster, "Instrument.lvclass"=w256:refnum<class "Instrument.lvclass">, "Instrument UI out"=w257:refnum<class "Instrument.Oxford1820 UI.lvclass">)  [unwired: 7 in]
            n100 = To More Specific Class(target class=w255, reference=w256) -> (specific class reference=w258:refnum<class "Instrument.Oxford1820.lvclass">)  [unwired: 1 in, 1 out]
            n101 = Get Date/Time In Seconds() -> (seconds since 1Jan1904=w266:timestamp)
            n102 = Variant To Data(error in=w259, type=w267, Variant=w266) -> (data=w264:timestamp, error out=w265:errorcluster)
            n103 = Bundle("Core"=w271, "Instrument UI out"=w257, "Instrument"=w258, "getAll"=w270, "Response"=w269, "config"=w268, "switch time"=w264, "LPF time"=w263) -> (w275:T9)  [unwired: 1 in]
            n104 = call <vilib>:"Add State(s) to Queue__jki_lib_state_machine.vi"("State(s) in (\"\")"=w277) -> ("States Out"=w276:string)  [unwired: 14 in]
          }
          frame "Data: Cleanup" {
            # "Cleanup any data and references, here.\n(this is called automatically, by the Macro: Exit)"
            n105 = Unbundle By Name(w279) -> ("Core.Current VI Reference"=w282:refnum<vi>)
            n106 = Close Reference(reference=w282, error in (no error)=w281) -> (error out=w280:errorcluster)
            n107 = call <vilib>:"Add State(s) to Queue__jki_lib_state_machine.vi"("State(s) in (\"\")"=w284) -> ("States Out"=w283:string)  [unwired: 14 in]
          }
          frame "---------- UI ----------" {
            # "Do not put any code in this frame.\n(It is a separator no-op. You can make a copy of this frame to create a new UI frame)"
            n108 = call <vilib>:"Add State(s) to Queue__jki_lib_state_machine.vi"("State(s) in (\"\")"=w289) -> ("States Out"=w288:string)  [unwired: 14 in]
          }
          frame "UI: Initialize" {
            # "size window to decoration box on front panel"
            # "Initialize the User Interface, here.\n(this is called automatically, by the Macro: Init)"
            n109 = property on="Window Minimize" class="Bool (strict)"("Value"=FALSE ("Window Maximize"), "Visible"=TRUE ("Window Maximize")) -> ()  [unwired: 2 in, 2 out]
            n110 = property on="Window Maximize" class="Bool (strict)"("Value"=FALSE ("Window Maximize"), "Visible"=FALSE ("Window Maximize")) -> ()  [unwired: 2 in, 2 out]
            n111 = invoke on="Power" class="Bool (strict)" method="Reinit To Default"() -> ()  [unwired: 3 in, 3 out]
            n112 = call <userlib>:"Fit VI window to Largest Dec__ogtk.vi"("error in (no error)"=w296, "border spacing (2 px)"=0) -> ("error out"=w295:errorcluster)  [unwired: 4 in, 1 out]
            n113 = call <vilib>:"Add State(s) to Queue__jki_lib_state_machine.vi"("State(s) in (\"\")"=w300) -> ("States Out"=w299:string)  [unwired: 14 in]
          }
          frame "UI: Update Front Panel All" {
            n114 = Unbundle By Name(w323) -> ("getAll"=w320:variant)
            n115 = Variant To Data(error in=w322, type=T4 {"1820_IPS_Magnet_Field"=0.0, "1820_IPS_PS_Field"=0.0, "1820_IPS_Target_Field"=0.0, "1820_IPS_Target_Field_Rate"=0.0, "1820_IPS_Voltage"=0.0, "1820_IPS_Current"=0.0, "1820_IPS_Level_N2"=0.0, "1820_IPS_Level_He"=0.0, "1820_IPS_Magnet_Temperature"=0.0, "1820_IPS_Magnet_Temperature_R"=0.0, "1820_IPS_M1_Current"=0.0, "1820_IPS_M1_Voltage"=0.0, "1820_IPS_M2_Current"=0.0, "1820_IPS_M2_Voltage"=0.0, "1820_IPS_M3_Current"=0.0, "1820_IPS_M3_Voltage"=0.0, "1820_IPS_Status"="", "1820_IPS_Switch"="", "1820_ITC_Lambda_Temperature"=0.0, "1820_ITC_Lambda_Temperature_R"=0.0, "1820_ITC_Pressure"=0.0, "1820_ITC_Needle_Valve"=0.0} ("getAll"), Variant=w320) -> (data=w318:T4, error out=w321:errorcluster)
            n116 = Unbundle By Name(w318) -> ("1820_IPS_Magnet_Field"=→"Field" →"Magnet Field Meter":dbl, "1820_IPS_PS_Field"=→"PSU Field":dbl, "1820_IPS_Target_Field"=→"Target Field (T)":dbl, "1820_IPS_Target_Field_Rate"=→"Target Rate (T/min)":dbl, "1820_IPS_Voltage"=→"Voltage" →"Voltage Meter":dbl, "1820_IPS_Current"=→"Current" →"Current Meter":dbl, "1820_IPS_Level_N2"=w303:dbl, "1820_IPS_Level_He"=w304:dbl, "1820_IPS_Status"=w305:string, "1820_IPS_Switch"=w302:string, "1820_ITC_Lambda_Temperature"=→"Magnet T":dbl, "1820_ITC_Lambda_Temperature_R"=→"Magnet R":dbl, "1820_ITC_Pressure"=→"Pressure":dbl, "1820_ITC_Needle_Valve"=→"Needle Valve":dbl)  [unwired: 8 out]
            "He LEVEL" <- w304
            "He LVL" <- w304
            "He LVL Chart" <- w304
            "N2 LVL Chart" <- w303
            "N2 LVL" <- w303
            "N2 LEVEL" <- w303
            n117 = call "Switch Status String to Boolean.vi"("String"=w302) -> ("Switch:"=w301:bool)
            n118 = call "Action Status to Text.vi"("PSU Act Stat"=w305) -> ("Status:"=→"Magnet Status 3":string)
            n119 = local write "PS Heat"(w301) -> ()
            n120 = Bundle("1820_IPS_Level_He"=w304, "1820_IPS_Level_N2"=w303) -> (→"Waveform Chart 2":T1)  [unwired: 1 in]
            n121 = call <vilib>:"Add State(s) to Queue__jki_lib_state_machine.vi"("State(s) in (\"\")"=w326) -> ("States Out"=w325:string)  [unwired: 14 in]
          }
          frame "UI: Update Front Panel Time" {
            # "Do not put any code in this frame.\n(It is a separator no-op. You can make a copy of this frame to create a new UI frame)"
            n122 = Unbundle By Name(w340) -> ("switch time"=w338:timestamp, "LPF time"=w337:timestamp)
            n123 = local read "LPF Power"() -> (w334:bool)
            n124 = Get Date/Time In Seconds() -> (seconds since 1Jan1904=w330:timestamp)
            n125 = local read "Target Rate (T/min)"() -> (w332:dbl)
            n126 = local read "Target Field (T)"() -> (w335:dbl)
            n127 = local read "PSU Field"() -> (w331:dbl)
            n128 = local read "Field"() -> (w333:dbl)
            n129 = To Double Precision Float(number=w330) -> (double precision float=→"System Time (HH:MM:SS)":dbl)
            n130 = call "1820 PS Heat duration.vi"("time stamp"=w338) -> ("PS Heat on (HH:MM:SS)"=→"PS Heat on (HH:MM:SS)":dbl)  [unwired: 10 in]
            n131 = call "1820 LPF ON duration.vi"("Lambda"=w334, "LPF ON"=w337) -> ("LPF on (HH:MM:SS)"=→"LPF on":dbl)  [unwired: 9 in]
            n132 = call "1820 Sweep ETA.vi"("Power Supply Field (T)"=w331, "Target Field Rate (T/min)"=w332, "Magnet Field (T)"=w333, "Target Field (T)"=w335) -> ("ETA timestamp"=w328:timestamp)  [unwired: 5 in, 2 out]
            n133 = To Double Precision Float(number=w328) -> (double precision float=→"ETA":dbl)
            n134 = call <vilib>:"Add State(s) to Queue__jki_lib_state_machine.vi"("State(s) in (\"\")"=w344) -> ("States Out"=w343:string)  [unwired: 14 in]
          }
          frame "UI: Status 2" {
            # "Do not put any code in this frame.\n(It is a separator no-op. You can make a copy of this frame to create a new UI frame)"
            n135 = call <vilib>:"Add State(s) to Queue__jki_lib_state_machine.vi"("State(s) in (\"\")"=w350) -> ("States Out"=w349:string)  [unwired: 14 in]
            "Magnet Status 2" <- w345
          }
          frame "UI: Level Colors" {
            # "Do not put any code in this frame.\n(It is a separator no-op. You can make a copy of this frame to create a new UI frame)"
            n136 = control-ref of="He LVL Chart"() -> (w352:refnum<vi>)
            n137 = call "Level Color.vi"("LVL Chart Refernce"=w352) -> ()  [unwired: 11 in]
            n138 = control-ref of="N2 LVL Chart"() -> (w351:refnum<vi>)
            n139 = call "Level Color.vi"("LVL Chart Refernce"=w351) -> ()  [unwired: 11 in]
            n140 = call <vilib>:"Add State(s) to Queue__jki_lib_state_machine.vi"("State(s) in (\"\")"=w357) -> ("States Out"=w356:string)  [unwired: 14 in]
          }
          frame "UI: Cursor Set" {
            # "Argument"
            # "Initialize the User Interface, here.\n(this is called automatically, by the Macro: Init)"
            n141 = disable-structure shown="Default" {
              disable-tunnel: w360 -> [w365 w368]
              disable-tunnel: [w365 w367] -> w359
              disable-tunnel: w358 -> [_ w366]
              frame condition #0 {
              }
              frame condition #1 (active) {
                n142 = case shown="\"Idle\", Default" w366 {
                  tunnel: w368 -> [w370 w372]
                  tunnel: [w369 w371] -> w367
                  frame "Idle", Default {
                    n143 = call <vilib>:"Unset Busy.vi"("error in (no error)"=w370) -> ("error out"=w369:errorcluster)  [unwired: 10 in]
                  }
                  frame "Busy" {
                    n144 = call <vilib>:"Set Busy.vi"("error in (no error)"=w372) -> ("error out"=w371:errorcluster)  [unwired: 9 in, 1 out]
                  }
                }
              }
            }
            n145 = call <vilib>:"Add State(s) to Queue__jki_lib_state_machine.vi"("State(s) in (\"\")"=w364) -> ("States Out"=w363:string)  [unwired: 14 in]
          }
          frame "UI: Front Panel State" {
            # "Argument"
            # "Set Front Panel Open or Closed\n(Usage: \"UI: Front Panel State >> Open|Close\")"
            n146 = Unbundle By Name(w376) -> ("Core.Current VI Reference"=w375:refnum<vi>)
            n147 = disable-structure shown="Default" {
              disable-tunnel: w378 -> [w384 w407]
              disable-tunnel: [w383 w407] -> w377
              disable-tunnel: w375 -> [w382 _]
              disable-tunnel: w374 -> [w381 _]
              frame condition #0 (active) {
                n148 = case shown="\"Close\"" w381 {
                  tunnel: w384 -> [w388 w401]
                  tunnel: [w390 w402] -> w383
                  tunnel: w382 -> [w389 w399]
                  frame "Open", Default {
                    n149 = property class="VI"(reference=w389, error in=w388) -> (reference out=w386:refnum<vi>, error out=w387:errorcluster, "FP.State"=w385:T5)
                    n150 = case shown="\"Closed\"" w385 {
                      tunnel: [w393 w396] -> w390
                      tunnel: w387 -> [w392 w396]
                      tunnel: w386 -> [w391 _]
                      frame "Closed" {
                        n151 = invoke class="VI" method="FP.Open"(reference=w391, error in=w392, "Activate"=TRUE, "State"=T5."Standard") -> (error out=w393:errorcluster)  [unwired: 1 in, 4 out]
                      }
                      frame Default {
                      }
                    }
                  }
                  frame "Close" {
                    n152 = property class="VI"(reference=w399, error in=w401) -> (reference out=w398:refnum<vi>, error out=w400:errorcluster, "FP.State"=w397:T5)
                    n153 = case shown="Default" w397 {
                      tunnel: [w403 w406] -> w402
                      tunnel: w400 -> [w403 w405]
                      tunnel: w398 -> [_ w404]
                      frame "Invalid", "Closed" {
                      }
                      frame Default {
                        n154 = invoke class="VI" method="FP.Close"(reference=w404, error in=w405) -> (error out=w406:errorcluster)  [unwired: 1 in, 2 out]
                      }
                    }
                  }
                }
              }
              frame condition #1 {
              }
            }
            n155 = call <vilib>:"Add State(s) to Queue__jki_lib_state_machine.vi"("State(s) in (\"\")"=w380) -> ("States Out"=w379:string)  [unwired: 14 in]
          }
          frame "UI: Minimize" {
            # "Do not put any code in this frame.\n(It is a separator no-op. You can make a copy of this frame to create a new UI frame)"
            n156 = Unbundle By Name(w413) -> ("Core.Current VI Reference"=w412:refnum<vi>)
            n157 = property class="VI"(reference=w412, error in=w409) -> (reference out=w411:refnum<vi>, error out=w410:errorcluster, "Front Panel.PanelBounds"=w417:T11)
            n158 = case shown="\"Min\", Default" w415 {
              tunnel: w417 -> [w420 w428]
              tunnel: [w427 w435] -> w416
              frame "Min", Default {
                n159 = Unbundle By Name(w420) -> ("Left"=w426:i16, "Top"=w424:i16)
                n160 = Add(x=i16 776 ("x 6"), y=w426) -> (x+y=w425:i16)
                n161 = Add(x=w424, y=i16 184 ("x 5")) -> (x+y=w423:i16)
                n162 = Bundle By Name(cluster=w420, "Right"=w425, "Bottom"=w423) -> (w427:T11)
              }
              frame "Max" {
                n163 = Unbundle By Name(w428) -> ("Left"=w434:i16, "Top"=w432:i16)
                n164 = Add(x=i16 1168 ("x 8"), y=w434) -> (x+y=w433:i16)
                n165 = Add(x=w432, y=i16 584 ("x 7")) -> (x+y=w431:i16)
                n166 = Bundle By Name(cluster=w428, "Right"=w433, "Bottom"=w431) -> (w435:T11)
              }
            }
            n167 = property class="VI"(reference=w411, error in=w410, "Front Panel.PanelBounds"=w416) -> (error out=w408:errorcluster)  [unwired: 1 out]
            n168 = call <vilib>:"Add State(s) to Queue__jki_lib_state_machine.vi"("State(s) in (\"\")"=w414) -> ("States Out"=w419:string)  [unwired: 14 in]
          }
          frame "---------- Macro ----------" {
            # "Do not put any code in this frame.\n(It is a separator no-op. You can make a copy of this frame to create a new Macro frame)"
            n169 = call <vilib>:"Add State(s) to Queue__jki_lib_state_machine.vi"("State(s) in (\"\")"=w440) -> ("States Out"=w439:string)  [unwired: 14 in]
          }
          frame "Macro: Initialize" {
            w443 = "UI: Initialize\nUI: Front Panel State >> Open\nUI: Status 2 >> ..."  # UI: Initialize UI: Front Panel State >> Open UI: Status 2 >> ...
            # "Initialization Macro\n(This is called once, when the VI starts)"
            n170 = call <vilib>:"Add State(s) to Queue__jki_lib_state_machine.vi"("State(s) in Front (\"\")"="Data: Initialize\nInitialize Core Data\nEvents: Register", "State(s) in (\"\")"="Process: Sync", "State(s) at Back (\"\")"=w443) -> ("States Out"=w442:string)  [unwired: 12 in]
            n171 = call <vilib>:"Add State(s) to Queue__jki_lib_state_machine.vi"("State(s) in Front (\"\")"=w442, "State(s) in (\"\")"=w449) -> ("States Out"=w448:string)  [unwired: 13 in]
          }
          frame "Macro: Exit" {
            # "Exit Macro\n(This is called once, when the VI exits)"
            n172 = Unbundle By Name(w454) -> ("Core.Close Panel on Exit?"=w460:bool)
            n173 = Select(t="UI: Front Panel State >> Close", s=w460, f="") -> (s? t:f=w457:string)
            n174 = call <vilib>:"Add State(s) to Queue__jki_lib_state_machine.vi"("State(s) in Front (\"\")"="Data: Cleanup\nEvents: Unregister\nProcess: Self Terminate", "State(s) in (\"\")"="Process: Sync", "State(s) at Back (\"\")"="Exit") -> ("States Out"=w451:string)  [unwired: 12 in]
            n175 = call <vilib>:"Add State(s) to Queue__jki_lib_state_machine.vi"("State(s) in (\"\")"=w457, "State(s) at Back (\"\")"=w451) -> ("States Out"=w456:string)  [unwired: 13 in]
            n176 = call <vilib>:"Add State(s) to Queue__jki_lib_state_machine.vi"("State(s) in Front (\"\")"=w456, "State(s) in (\"\")"=w463) -> ("States Out"=w462:string)  [unwired: 13 in]
          }
          frame "---------- Process ----------" {
            # "Template Separator\n(You can make a copy of, or modify, this frame)"
            n177 = call <vilib>:"Add State(s) to Queue__jki_lib_state_machine.vi"("State(s) in (\"\")"=w468) -> ("States Out"=w467:string)  [unwired: 14 in]
          }
          frame "Process: Sync" {
            n178 = Unbundle By Name(w476) -> ("Instrument UI out"=w472:refnum<class "Instrument.Oxford1820 UI.lvclass">)
            n179 = call <vilib>:"WaitOnProcessSync.vi"("error in (no error)"=w471, "SMO"=w472) -> ("error out"=w470:errorcluster, "Don't run?"=w475:bool)  [unwired: 7 in, 1 out]
            n180 = Select(t="Data: Cleanup\nEvents: Unregister\nExit", s=w475, f="") -> (s? t:f=w469:string)
            n181 = call <vilib>:"Add State(s) to Queue__jki_lib_state_machine.vi"("State(s) in Front (\"\")"=w469, "State(s) in (\"\")"=w479) -> ("States Out"=w478:string)  [unwired: 13 in]
          }
          frame "Process: Self Terminate" {
            n182 = Unbundle By Name(w481) -> ("Instrument UI out"=w480:refnum<class "Instrument.Oxford1820 UI.lvclass">)
            n183 = call <vilib>:"SelfTerminate.vi"("error in (no error)"=w483, "SMO in"=w480) -> ("error out"=w482:errorcluster)  [unwired: 8 in, 1 out]
            n184 = call <vilib>:"Add State(s) to Queue__jki_lib_state_machine.vi"("State(s) in (\"\")"=w486) -> ("States Out"=w485:string)  [unwired: 14 in]
          }
          frame "---------- Events ----------" {
            # "Template Separator\n(You can make a copy of, or modify, this frame)"
            n185 = call <vilib>:"Add State(s) to Queue__jki_lib_state_machine.vi"("State(s) in (\"\")"=w491) -> ("States Out"=w490:string)  [unwired: 14 in]
          }
          frame "Events: Register" {
            # "Expand to add\nmore events"
            # "Base Class Protected Events"
            n186 = Unbundle By Name(w503) -> ("Instrument UI out"=w497:refnum<class "Instrument.Oxford1820 UI.lvclass">, "Instrument"=w495:refnum<class "Instrument.Oxford1820.lvclass">)
            n187 = call <vilib>:"GetProtectedEvents.vi"("SMO"=w497) -> ("error out"=w498:errorcluster, "SMO Protected Events"=w501:T12)  [unwired: 8 in, 1 out]
            n188 = call <userlib>:"Instrument.GetPublicEvents.vi"("Instrument"=w495) -> ("error out"=w496:errorcluster, "Instrument Public Events"=w492:T13, "Instrument out"=w493:refnum<class "Instrument.Oxford1820.lvclass">)  [unwired: 8 in]
            n189 = flat-sequence {
              tunnel: w493 -> [_]
              frame #0 {
              }
            }
            n190 = register-events(w501, w492) -> (reference out=w502:refnum<event-registration>, error out=w500:errorcluster)  [unwired: 2 in]
            n191 = Merge Errors(w496, w494, w500, w498) -> (w499:errorcluster)
            n192 = call <vilib>:"Add State(s) to Queue__jki_lib_state_machine.vi"("State(s) in (\"\")"=w505) -> ("States Out"=w504:string)  [unwired: 14 in]
          }
          frame "Events: Unregister" {
            n193 = Unregister For Events(event registration refnum=w508, error in=w507) -> (error out=w506:errorcluster)
            n194 = call <vilib>:"Add State(s) to Queue__jki_lib_state_machine.vi"("State(s) in (\"\")"=w511) -> ("States Out"=w510:string)  [unwired: 14 in]
          }
          frame "---------- Action ----------" {
            n195 = Unbundle By Name(w514) -> ("Instrument UI out"=w512:refnum<class "Instrument.Oxford1820 UI.lvclass">)
            n196 = Bundle By Name(cluster=w514, "Instrument UI out"=w512) -> (w513:T9)
            n197 = call <vilib>:"Add State(s) to Queue__jki_lib_state_machine.vi"("State(s) in (\"\")"=w518) -> ("States Out"=w517:string)  [unwired: 14 in]
          }
          frame "Action: Notify UI Closed" {
            # "Notify that the UI has been closed"
            n198 = Unbundle By Name(w521) -> ("Instrument UI out"=w522:refnum<class "Instrument.Oxford1820 UI.lvclass">)
            n199 = call <vilib>:"Hide.vi"("error in (no error)"=w520, "SMO.UI"=w522) -> ("error out"=w519:errorcluster)  [unwired: 8 in, 1 out]
            n200 = call <vilib>:"Add State(s) to Queue__jki_lib_state_machine.vi"("State(s) in (\"\")"=w525) -> ("States Out"=w524:string)  [unwired: 14 in]
          }
          frame "Action: get All" {
            n201 = Unbundle By Name(w526) -> ("Instrument"=w531:refnum<class "Instrument.Oxford1820.lvclass">)
            n202 = call <userlib>:"Get ALL.vi"("error in (no error)"=w530, "Instrument in"=w531) -> ("error out"=w529:errorcluster, "getAll"=w527:variant, "Instrument out"=w528:refnum<class "Instrument.Oxford1820.lvclass">)  [unwired: 7 in]
            n203 = Bundle By Name(cluster=w526, "Instrument"=w528, "getAll"=w527) -> (w532:T9)
            n204 = call <vilib>:"Add State(s) to Queue__jki_lib_state_machine.vi"("State(s) in (\"\")"=w535) -> ("States Out"=w534:string)  [unwired: 14 in]
          }
          frame "Action: Hold" {
            n205 = Unbundle By Name(w539) -> ("Instrument"=w538:refnum<class "Instrument.Oxford1820.lvclass">)
            n206 = call "Hold.vi"("error in (no error)"=w537, "Instrument.1820 in"=w538) -> ("error out"=w536:errorcluster)  [unwired: 7 in, 2 out]
            n207 = call <vilib>:"Add State(s) to Queue__jki_lib_state_machine.vi"("State(s) in (\"\")"=w542) -> ("States Out"=w541:string)  [unwired: 14 in]
          }
          frame "Action: To Zero" {
            n208 = Unbundle By Name(w546) -> ("Instrument"=w545:refnum<class "Instrument.Oxford1820.lvclass">)
            n209 = call "Ramp to Zero.vi"("error in (no error)"=w544, "Instrument.1820 in"=w545) -> ("error out"=w543:errorcluster)  [unwired: 7 in, 2 out]
            n210 = call <vilib>:"Add State(s) to Queue__jki_lib_state_machine.vi"("State(s) in (\"\")"=w549) -> ("States Out"=w548:string)  [unwired: 14 in]
          }
          frame "Action: To Set" {
            n211 = Unbundle By Name(w553) -> ("Instrument"=w552:refnum<class "Instrument.Oxford1820.lvclass">)
            n212 = call "Ramp to Set.vi"("error in (no error)"=w551, "Instrument.1820 in"=w552) -> ("error out"=w550:errorcluster)  [unwired: 7 in, 2 out]
            n213 = call <vilib>:"Add State(s) to Queue__jki_lib_state_machine.vi"("State(s) in (\"\")"=w556) -> ("States Out"=w555:string)  [unwired: 14 in]
          }
          frame "Action: Clamp" {
            n214 = Unbundle By Name(w557) -> ("Instrument"=w560:refnum<class "Instrument.Oxford1820.lvclass">)
            n215 = call "Clamp.vi"("error in (no error)"=w559, "Instrument.1820 in"=w560) -> ("error out"=w558:errorcluster)  [unwired: 7 in, 2 out]
            n216 = call <vilib>:"Add State(s) to Queue__jki_lib_state_machine.vi"("State(s) in (\"\")"=w563) -> ("States Out"=w562:string)  [unwired: 14 in]
          }
          frame "Action: Fill" {
            n217 = Unbundle By Name(w571) -> ("Instrument"=w570:refnum<class "Instrument.Oxford1820.lvclass">)
            n218 = Select(t=T6 "OFF" ("Fill Mode"), s="Fast/Slow Fill", f=T6 "ON" ("Fill Mode")) -> (s? t:f=w566:T6)
            n219 = call "Set Fill Mode.vi"("error in (no error)"=w569, "Fill Mode"=w566, "Instrument.1820 in"=w570) -> ("error out"=w568:errorcluster)  [unwired: 6 in, 2 out]
            n220 = call <vilib>:"Add State(s) to Queue__jki_lib_state_machine.vi"("State(s) in (\"\")"=w574) -> ("States Out"=w573:string)  [unwired: 14 in]
          }
          frame "Action: LPF" {
            n221 = Unbundle By Name(w577) -> ("Instrument"=w584:refnum<class "Instrument.Oxford1820.lvclass">)
            n222 = Select(t=T7 "ON" ("LPF State"), s="LPF Power", f=T7 "OFF" ("LPF State")) -> (s? t:f=w581:T7)
            n223 = call "Set LPF State.vi"("error in (no error)"=w583, "LPF State"=w581, "Instrument.1820 in"=w584) -> ("error out"=w582:errorcluster)  [unwired: 6 in, 2 out]
            n224 = Get Date/Time In Seconds() -> (seconds since 1Jan1904=w575:timestamp)
            n225 = Bundle By Name(cluster=w577, "LPF time"=w575) -> (w576:T9)
            n226 = call <vilib>:"Add State(s) to Queue__jki_lib_state_machine.vi"("State(s) in (\"\")"=w587) -> ("States Out"=w586:string)  [unwired: 14 in]
          }
          frame "Action: Needle Valve" {
            # "2=open"
            # "1=closed"
            n227 = Unbundle By Name(w597) -> ("Instrument"=w596:refnum<class "Instrument.Oxford1820.lvclass">)
            n228 = Build Array("Close Needle Valve", "Open Needle Valve") -> (w594:bool[])
            n229 = Boolean Array To Number(Boolean array=w594) -> (number=w591:u32)
            n230 = case shown="1, Default" w591 {
              tunnel: [0.0 ("Needle Valve (%)") "Open Target"] -> w590
              frame 1, Default {
              }
              frame 2 {
              }
            }
            n231 = call "Set Needle Valve.vi"("error in (no error)"=w595, "Needle Valve (%)"=w590, "Instrument.1820 in"=w596) -> ("error out"=w589:errorcluster)  [unwired: 6 in, 2 out]
            n232 = flat-sequence {
              tunnel: [w601] -> w588
              tunnel: w589 -> [w601]
              frame #0 {
                n233 = local write "Close Needle Valve"(FALSE ("Close Needle Valve")) -> ()
                n234 = local write "Open Needle Valve"(FALSE ("Open Needle Valve")) -> ()
              }
            }
            n235 = call <vilib>:"Add State(s) to Queue__jki_lib_state_machine.vi"("State(s) in (\"\")"=w600) -> ("States Out"=w599:string)  [unwired: 14 in]
          }
          frame "Action: PS Heat" {
            n236 = Unbundle By Name(w609) -> ("Instrument"=w606:refnum<class "Instrument.Oxford1820.lvclass">)
            n237 = Select(t=T7 "ON" ("LPF State"), s="PS Heat", f=T7 "OFF" ("LPF State")) -> (s? t:f=w613:T7)
            n238 = call "Set Switch Heater.vi"("error in (no error)"=w615, "Switch Heater"=w613, "Instrument.1820 in"=w606) -> ("error out"=w614:errorcluster)  [unwired: 6 in, 2 out]
            n239 = Get Date/Time In Seconds() -> (seconds since 1Jan1904=w608:timestamp)
            n240 = Bundle By Name(cluster=w609, "switch time"=w608) -> (w607:T9)
            n241 = call <vilib>:"Add State(s) to Queue__jki_lib_state_machine.vi"("State(s) in (\"\")"=w618) -> ("States Out"=w617:string)  [unwired: 14 in]
          }
          frame "Action: Send to IPS" {
            n242 = Unbundle By Name(w624) -> ("Instrument"=w623:refnum<class "Instrument.Oxford1820.lvclass">)
            n243 = call "Set Target.vi"("error in (no error)"=w622, "Target Rate (T/min)"="Target Rate (T/min)", "Target Field (T)"="Target Field (T)", "Instrument.1820 in"=w623) -> ("error out"=w621:errorcluster)  [unwired: 5 in, 2 out]
            n244 = call <vilib>:"Add State(s) to Queue__jki_lib_state_machine.vi"("State(s) in (\"\")"=w627) -> ("States Out"=w626:string)  [unwired: 14 in]
          }
        }
      }
    }
    frame Error {
    }
  }
  n245 = call-parent "Process.vi"("error in"=w9, "Instrument UI in"=w8) -> ("error out"=w6:errorcluster, "Instrument UI out"=→"Oxford1820 UI out":refnum<class "Instrument.Oxford1820 UI.lvclass">)  [unwired: 8 in]
  n246 = disable-structure shown="Disabled" {
    frame Disabled {
    }
    frame Enabled {
    }
  }
  n247 = Merge Errors(w6, w5) -> (→"error out":errorcluster)
  "version" <- "v20/12/08" ("version")
